vi "HTL parameters.vi"(4 "Move on":bool, 6 "Tab Control":enum32{"Fixed Steps", "Free Style Steps"}(tab), 7 "RampSelect":bool[](array[boolean])=[TRUE, TRUE, FALSE, FALSE, FALSE, FALSE], 8 "Maximum Allowed Field":dbl=99.0 format="%.2f", 9 "File Path Para Array":T1[](array[typedef]), 10 "#Points":u32[](array[numeric])=[30, 30, 30, 30, 60, 60] step=1, 11 "FieldRamp Parameters":dbl[][](array[numeric])=[[0.0, 30.0, 1.0, 20.0], [30.0, 0.0, -1.0, 20.0], [0.0, -30.0, -1.0, 20.0], [-30.0, 0.0, 1.0, 20.0], [0.0, 30.0, 0.5, 20.0], [30.0, 0.0, -0.5, 20.0]] step=1.0 format="%.2f") -> (0 "HTL Array":dbl[][](array[numeric]), 1 "Path array":path[](array[path]), 2 "Prefix Indexed output":bool, 3 "SubFolderNamesArray":string[](array[string]))   [LabVIEW 2020]
uses:
  Globals and TypeDefs/Type Definitions.llb/FilePathParameter.ctt
panel:
  in  "Prefix Indexed":bool=TRUE
  in  "Subfolder Names":string[](array[string])=["", "", "", "", "", " "]
  in  "Temperature Ramp Parameters":dbl[][](array[numeric])=[[-1.0, -1.0, 1.0, 20.0], [-1.0, -1.0, -1.0, 20.0], [-1.0, -1.0, -1.0, 20.0], [-1.0, -1.0, 1.0, 20.0], [-1.0, -1.0, 0.5, 20.0], [-1.0, -1.0, -0.5, 20.0]] step=1.0 format="%.2f"
  in  "Wavelength ramp Parameters":dbl[][](array[numeric])=[[-1.0, -1.0, 1.0, 20.0], [-1.0, -1.0, -1.0, 20.0], [-1.0, -1.0, -1.0, 20.0], [-1.0, -1.0, 1.0, 20.0], [-1.0, -1.0, 0.5, 20.0], [-1.0, -1.0, -0.5, 20.0]] step=1.0 format="%.2f"
  in  "SubFolder Name":string
  in  "Calcualte":bool caption="From the Fixed Steps?"
  in  "Temperature (K)":string
  in  "Wavelength":string
  in  "Field":string
  # "l (nm)"
  # "H(T)"
  # "T(K)"
  # "Select |#Points                 Hstart          Hend"
  # "l start                 l end"
  # "Subfolder"
  # "Tstart(K)   Tend(K)"
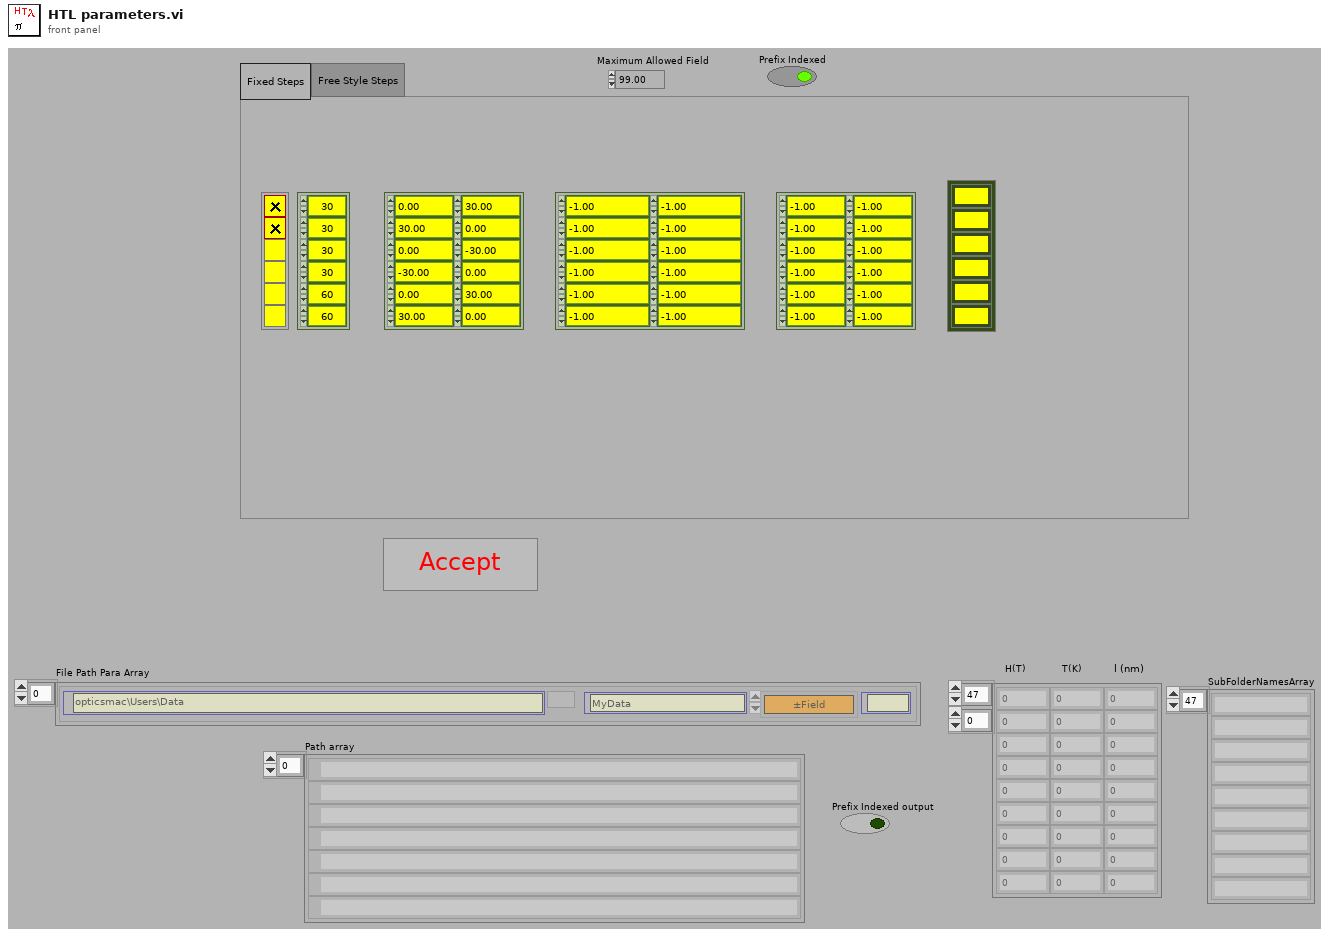
[diagram p1: front panel]
types:
  T1 = typedef "FilePathParameter.ctt" = cluster{"Filename Prefix":string, "Extension":enum16{"none", "\".001\",\".002\", ...", "001 (No dot)", "±Field", "pField nField", "Temperature", "Wavelength", "T(K)±H(T)", "(nm)T(K)±H(T)", "User Defined"}, "Suffix":string, "Current Path":path}
  T2 = enum8{"Field Step to #Points", "#Points to Field Steps"}
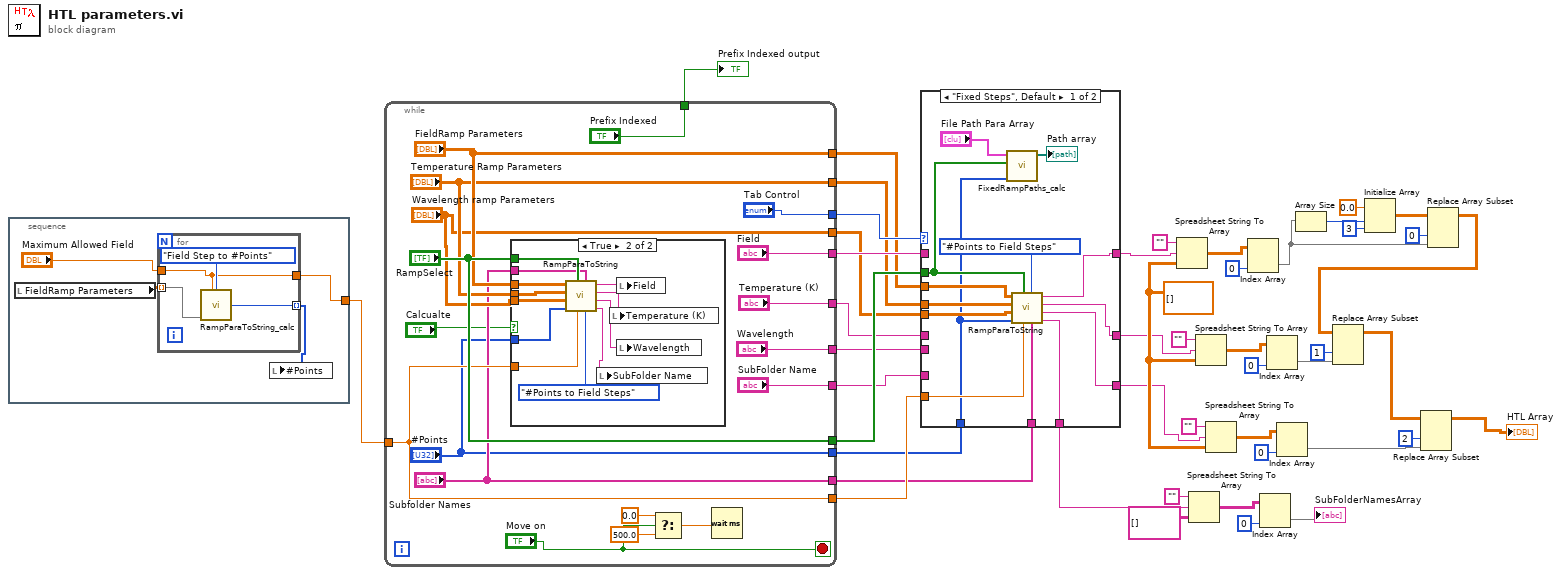
[diagram p0: block diagram]
diagram:
  w25 = dbl[][] [] ("array type (2D Dbl)")
  n1 = stacked-sequence {
    tunnel: [w48] -> w2
    frame #0 {
      n2 = local read "FieldRamp Parameters"() -> (w50:dbl[][])
      n3 = for {
        tunnel: w50 -> [w54] mode=indexing
        tunnel: [w52] -> w47 mode=indexing
        tunnel: "Maximum Allowed Field" -> [w51]
        tunnel: [w51] -> w48
        n4 = call "RampParaToString_calc.vi"("Mode"=T2."Field Step to #Points", "RampParameter"=w54, "Maximum Allowed Current"=w51) -> ("#Points output"=w52:u32)  [unwired: 2 in, 2 out]
      }
      n5 = local write "#Points"(w47) -> ()
    }
  }
  n6 = while {
    tunnel: w2 -> [w68]
    tunnel: ["Field"] -> w22
    tunnel: ["Tab Control"] -> w23
    tunnel: ["RampSelect"] -> w20
    tunnel: ["FieldRamp Parameters"] -> w19
    tunnel: [w68] -> w18
    tunnel: ["Temperature Ramp Parameters"] -> w17
    tunnel: ["Wavelength ramp Parameters"] -> w16
    tunnel: ["Temperature (K)"] -> w15
    tunnel: ["Wavelength"] -> w14
    tunnel: ["SubFolder Name"] -> w11
    tunnel: ["Subfolder Names"] -> w10
    tunnel: ["#Points"] -> w9
    tunnel: ["Prefix Indexed"] -> w1
    stop <- "Move on" stop-if-true
    n7 = case shown="True" "Calcualte" {
      tunnel: "RampSelect" -> [_ w84]
      tunnel: "FieldRamp Parameters" -> [_ w83]
      tunnel: w68 -> [_ w82]
      tunnel: "Temperature Ramp Parameters" -> [_ w81]
      tunnel: "Wavelength ramp Parameters" -> [_ w80]
      tunnel: "Subfolder Names" -> [_ w79]
      tunnel: "#Points" -> [_ w78]
      frame False {
      }
      frame True {
        n8 = call "RampParaToString.vi"("Mode"=T2."#Points to Field Steps", "Subfolder Names"=w79, "Maximum Allowed Current"=w82, "RampSelect"=w84, "#Points"=w78, "WavelengthRamp Parameters"=w80, "TempRamp Parameters"=w81, "FieldRamp Parameters"=w83) -> ("Subfolder strings"=w74:string, "Wavelength"=w75:string, "Temperature"=w76:string, "Field"=w77:string)
        n9 = local write "SubFolder Name"(w74) -> ()
        n10 = local write "Temperature (K)"(w76) -> ()
        n11 = local write "Field"(w77) -> ()
        n12 = local write "Wavelength"(w75) -> ()
      }
    }
    n13 = Select(t=0.0, s="Move on", f=500.0) -> (s? t:f=w58:dbl)
    n14 = Wait (ms)(milliseconds to wait=w58) -> ()  [unwired: 1 out]
  }
  "Prefix Indexed output" <- w1
  n15 = case shown="\"Fixed Steps\", Default" w23 {
    tunnel: [w96 w102] -> w21
    tunnel: w22 -> [_ w102]
    tunnel: w20 -> [w88 _]
    tunnel: w19 -> [w98 _]
    tunnel: w18 -> [w97 _]
    tunnel: w17 -> [w95 _]
    tunnel: w16 -> [w94 _]
    tunnel: w15 -> [_ w101]
    tunnel: w14 -> [_ w100]
    tunnel: [w93 w101] -> w13
    tunnel: [w92 w100] -> w12
    tunnel: w11 -> [_ w99]
    tunnel: w10 -> [w91 _]
    tunnel: w9 -> [w87 _]
    tunnel: [w90 w99] -> w8
    frame "Fixed Steps", Default {
      n16 = call "FixedRampPaths_calc.vi"("#Points"=w87, "RampSelect"=w88, "File Path Para Array out"="File Path Para Array") -> ("Path array"=→"Path array":path[])  [unwired: 4 in]
      n17 = call "RampParaToString.vi"("Mode"=T2."#Points to Field Steps", "Subfolder Names"=w91, "Maximum Allowed Current"=w97, "RampSelect"=w88, "#Points"=w87, "WavelengthRamp Parameters"=w94, "TempRamp Parameters"=w95, "FieldRamp Parameters"=w98) -> ("Subfolder strings"=w90:string, "Wavelength"=w92:string, "Temperature"=w93:string, "Field"=w96:string)
    }
    frame "Free Style Steps" {
    }
  }
  n18 = Spreadsheet String To Array(format string="", spreadsheet string=w21, array type (2D Dbl)=w25) -> (array=w27:dbl[][])  [unwired: 1 in]
  n19 = Spreadsheet String To Array(format string="", spreadsheet string=w8, array type (2D Dbl)=string[][] []) -> (array=w4:string[][])  [unwired: 1 in]
  n20 = Spreadsheet String To Array(format string="", spreadsheet string=w13, array type (2D Dbl)=w25) -> (array=w30:dbl[][])  [unwired: 1 in]
  n21 = Spreadsheet String To Array(format string="", spreadsheet string=w12, array type (2D Dbl)=w25) -> (array=w33:dbl[][])  [unwired: 1 in]
  n22 = Index Array(array=w27, index (col)=0 ("disabled index (col)")) -> (element=w40:dbl[])  [unwired: 1 in]
  n23 = Index Array(array=w4, index (col)=0 ("disabled index (col)")) -> (element=→"SubFolderNamesArray":string[])  [unwired: 1 in]
  n24 = Index Array(array=w30, index (col)=0 ("disabled index (col)")) -> (element=w43:dbl[])  [unwired: 1 in]
  n25 = Index Array(array=w33, index (col)=0 ("disabled index (col)")) -> (element=w45:dbl[])  [unwired: 1 in]
  n26 = Array Size(array=w40) -> (size(s)=w35:i32)
  n27 = Initialize Array(0.0 ("element"), w35, 3 ("dimension size")) -> (w38:dbl[][])
  n28 = Replace Array Subset(array=w38, new element=w40, index (col)=0 ("disabled index (col)")) -> (w46:dbl[][])  [unwired: 1 in]
  n29 = Replace Array Subset(array=w46, new element=w43, index (col)=1 ("disabled index (col)")) -> (w44:dbl[][])  [unwired: 1 in]
  n30 = Replace Array Subset(array=w44, new element=w45, index (col)=2 ("disabled index (col)")) -> (→"HTL Array":dbl[][])  [unwired: 1 in]
